vi "Get Notification Value.vi"(9 "notification in":cluster{"value":variant, "name":string}) -> (2 "data":variant, 3 "notification out":cluster{"value":variant, "name":string})   [LabVIEW 2014, in "Observable Actor.lvlib" / "Observable Actor.lvclass"]
uses:
  Observable Actor.lvclass
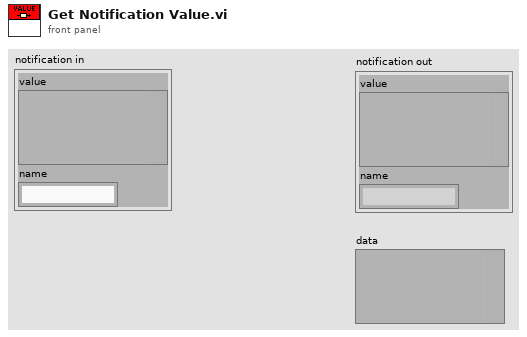
[diagram p1: front panel]
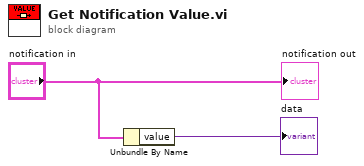
[diagram p0: block diagram]
diagram:
  n1 = Unbundle By Name("notification in") -> ("value"=→"data":variant)
  "notification out" <- "notification in"
